vi "colour_out-of-range_pixels.vi"(6 "colour":u32(colorbox)=16860, 8 "error in (no error)":errorcluster, 9 "comparison operator":T1, 10 "comparison value":dbl, 11 "Image in":refnum<class "Image.lvclass">) -> (0 "error out":errorcluster, 3 "Image out":refnum<class "Image.lvclass">)   [LabVIEW 2010, in "Image.lvclass"]
uses:
  Image.lvclass
  comparison_operator_enum.ctl
  ErrorController/ErrorController/class_data.vi
  ErrorController/ErrorController/ErrorController.lvclass
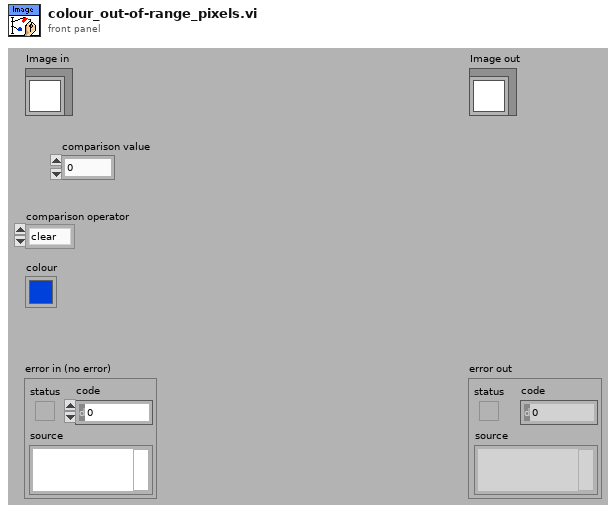
[diagram p1: front panel]
types:
  T1 = typedef "comparison_operator_enum.ctl" = enum16{"clear", "<", "=<", ">", "=>", "="}
  T2 = typedef "IMAQ Image.ctl" = refnum<image>
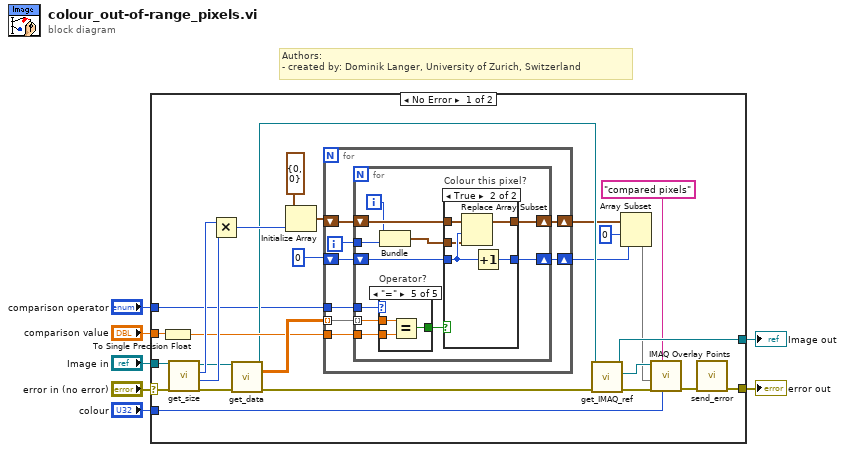
[diagram p0: block diagram]
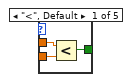
[diagram p2: hidden frame]
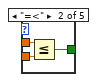
[diagram p3: hidden frame]
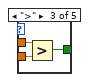
[diagram p4: hidden frame]
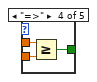
[diagram p5: hidden frame]
diagram:
  # "Authors: \n- created by: Dominik Langer, University of Zurich, Switzerland"
  n1 = case shown="No Error" "error in (no error)" {
    selector: "error in (no error)" -> [w32 w77]
    tunnel: [w8 w77] -> w6
    tunnel: [w19 w76] -> w4
    tunnel: "Image in" -> [w26 w76]
    tunnel: "comparison value" -> [w24 _]
    tunnel: "colour" -> [w18 _]
    tunnel: "comparison operator" -> [w17 _]
    frame No Error {
      n2 = To Single Precision Float(number=w24) -> (single precision float=w23:sgl)
      n3 = call-dynamic "get_size.vi"("error in (no error)"=w32, "Image in"=w26) -> ("error out"=w31:errorcluster, "y resolution"=w27:i32, "x resolution"=w28:i32, "Image out"=w25:refnum<class "Image.lvclass">)  [unwired: 2 in, 4 out]
      n4 = Multiply(x=w28, y=w27) -> (x*y=w29:i32)
      n5 = call-dynamic "get_data.vi"("Image in"=w25, "error in (no error)"=w31) -> ("Image out"=w20:refnum<class "Image.lvclass">, "Image Pixels (Float)"=w34:sgl[][], "error out"=w11:errorcluster)  [unwired: 5 in, 6 out]
      n6 = Initialize Array(cluster{"X":i32, "Y":i32} {"X"=0, "Y"=0} ("Point Coordinates"), w29) -> (w33:cluster{"X":i32, "Y":i32}[])
      n7 = for {
        tunnel: w34 -> [w42] mode=indexing
        shift-right: [w40] -> w16
        shift-left: w33 -> [w41]
        tunnel: w23 -> [w39]
        shift-right: [w37] -> w12
        shift-left: 0 -> [w38]
        tunnel: w17 -> [w35]
        i -> [w36]
        n8 = for {
          tunnel: w42 -> [w53] mode=indexing
          shift-right: [w47] -> w40
          shift-left: w41 -> [w51]
          tunnel: w39 -> [w52]
          shift-right: [w49] -> w37
          shift-left: w38 -> [w50]
          tunnel: w36 -> [w43]
          tunnel: w35 -> [w45]
          i -> [w44]
          n9 = case "Operator?" shown="\"=\"" w45 {
            tunnel: w53 -> [w56 w59 w62 w63 w67]
            tunnel: w52 -> [w55 w58 w61 w64 w68]
            tunnel: [w54 w57 w60 w65 w66] -> w48
            frame "<", Default {
              n10 = Less?(x=w56, y=w55) -> (x < y?=w54:bool)
            }
            frame "=<" {
              n11 = Less Or Equal?(x=w59, y=w58) -> (x <= y?=w57:bool)
            }
            frame ">" {
              n12 = Greater?(x=w62, y=w61) -> (0:w60:bool)
            }
            frame "=>" {
              n13 = Greater Or Equal?(x=w63, y=w64) -> (x >= y?=w65:bool)
            }
            frame "=" {
              n14 = Equal?(x=w67, y=w68) -> (x = y?=w66:bool)
            }
          }
          n15 = Bundle(w44, w43) -> (w46:cluster{i32, i32})  [unwired: 1 in]
          n16 = case "Colour this pixel?" shown="True" w48 {
            tunnel: w51 -> [w70 w75]
            tunnel: w50 -> [w69 w72]
            tunnel: [w69 w74] -> w49
            tunnel: [w70 w73] -> w47
            tunnel: w46 -> [_ w71]
            frame False {
            }
            frame True {
              n17 = Replace Array Subset(array=w75, new element=w71, index=w72) -> (w73:cluster{"X":i32, "Y":i32}[])
              n18 = Increment(x=w72) -> (x+1=w74:i32)
            }
          }
        }
      }
      n19 = call-dynamic "get_IMAQ_ref.vi"("error in (no error)"=w11, "Image.lvclass in"=w20) -> ("error out"=w13:errorcluster, "Image"=w21:T2, "Image.lvclass out"=w19:refnum<class "Image.lvclass">)  [unwired: 5 in, 2 out]
      n20 = Array Subset(array=w16, index=0, length=w12) -> (w15:cluster{"X":i32, "Y":i32}[])
      n21 = call "IMAQ Overlay Points"("Color"=w18, "Group"="compared pixels", "error in (no error)"=w13, "Array of Points"=w15, "Image"=w21) -> ("error out"=w9:errorcluster)  [unwired: 5 in, 1 out]
      n22 = call "send_error.vi"("error in (no error)"=w9) -> ("error out"=w8:errorcluster)  [unwired: 10 in]
    }
    frame Error {
    }
  }
  "error out" <- w6
  "Image out" <- w4
